vi "Test.vi"() -> ()   [LabVIEW 2016]
uses:
  Globals/PressuresGlobal.vi
  <userlib>/Fluigent/Fluigent MFCS/FluigentMFCS_Full.llb/MFCS_EZ Detect.vi
  <userlib>/Fluigent/Fluigent MFCS/FluigentMFCS_Full.llb/MFCS_EZ Initialization.vi
  <userlib>/Fluigent/Fluigent MFCS/FluigentMFCS_Full.llb/MFCS_EZ Write Channel Pressure.vi
  <vilib>/Utility/file.llb/Write Delimited Spreadsheet (DBL).vi
panel:
  out "Set Pressure Out 2":dbl[](array[numeric])=[825.7187370828326, 752.1790107184136]
  in  "Set Pressure in":dbl[](array[numeric])=[700.0, 700.0]
  out "Set Pressure Out":dbl[](array[numeric])
  in  "file path (dialog if empty)":path=path "E:/maggot images/Jacob/20180102/flow_across_channels_with_same_controller_run101.txt"
  out "Waveform Chart":T1(graph)={"appended array[0]"=534.7139256540268, "appended array[1]"=395.09418314500516}
  in  "Flowboards 2":enum16{"A", "B", "C"}[](array[ring])=[enum."A", enum."A", enum."A", enum."A", enum."B", enum."B"]
  in  "Channels 2":enum16{"1", "2", "3", "4", "5", "6", "7", "8"}[](array[ring])=[enum."1", enum."2", enum."3", enum."4", enum."1", enum."2"]
  in  "Channels":enum16{"1", "2", "3", "4", "5", "6", "7", "8"}[](array[ring])=[enum."1", enum."5"]
  in  "Flowboards":enum16{"A", "B", "C"}[](array[ring])=[enum."A", enum."A"]
  in  "Valve Data":T2
  in  "Water Mix Pressure Channel":i16=2
  in  "Odor Mix Pressure Channel":i16=3
  in  "Ratio":dbl=0.9
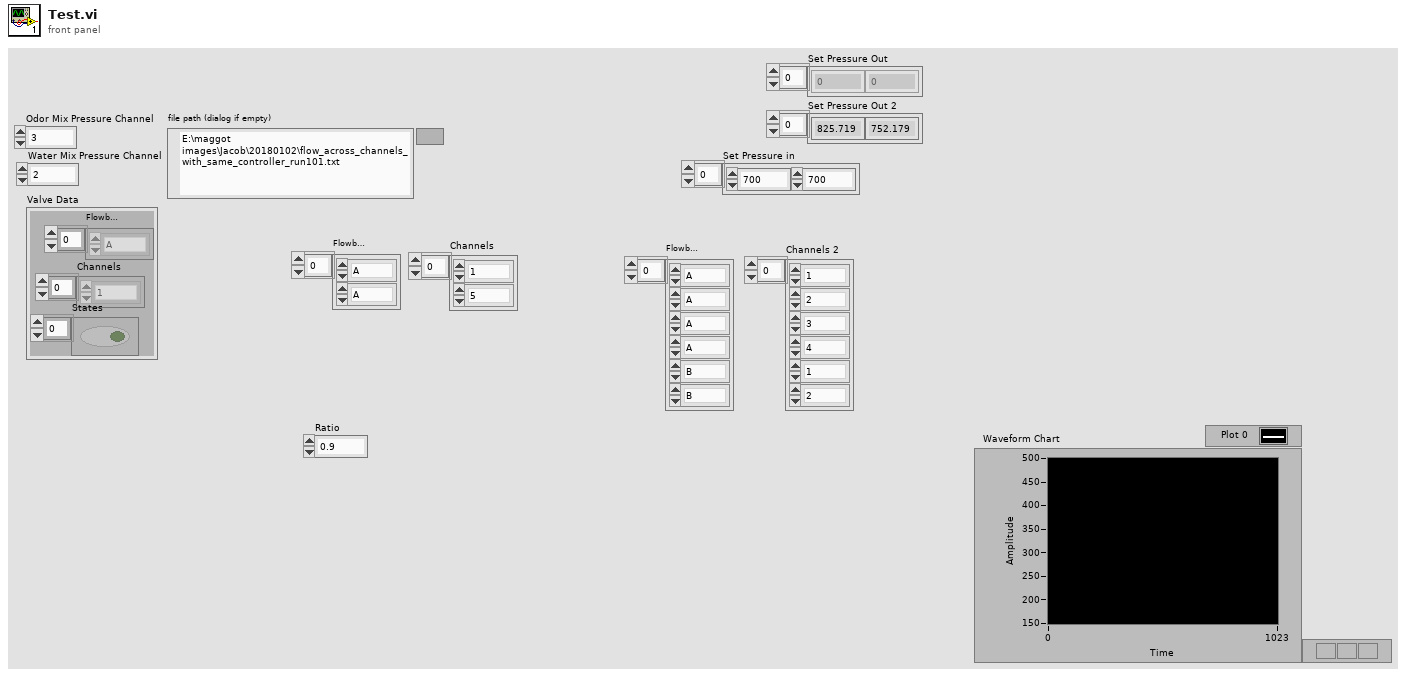
[diagram p1: front panel]
types:
  T1 = cluster{"appended array[0]":dbl, "appended array[1]":dbl}
  T2 = cluster{"Flowboards":enum16{"A", "B", "C"}[], "Channels":enum16{"1", "2", "3", "4", "5", "6", "7", "8"}[], "States":bool[]}
  T3 = enum16{"Release", "Create", "Send", "Wait", "Cancel"}
  T4 = typedef "_EZmfcsSN.ctl" = u16
  T5 = typedef "_EZmfcsRefNum.ctl" = refnum<k1>
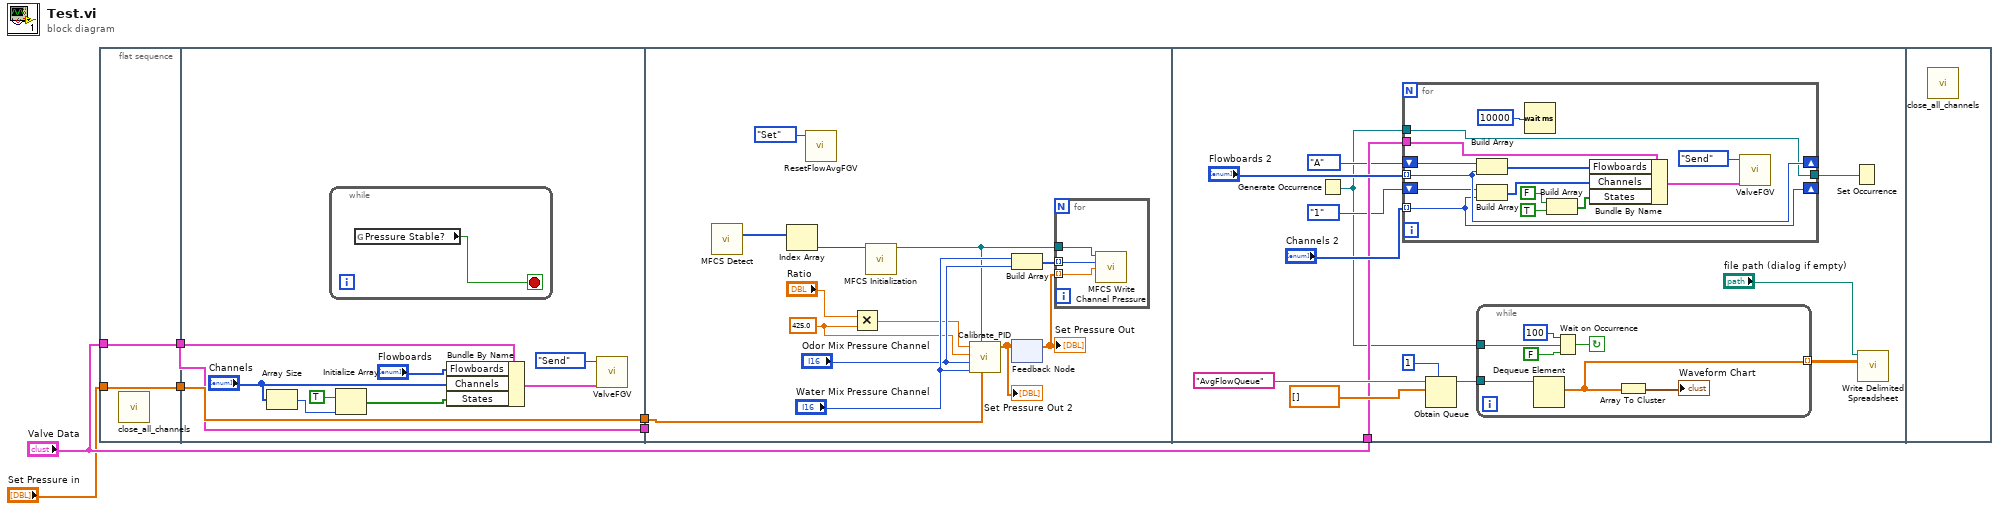
[diagram p0: block diagram]
diagram:
  n1 = flat-sequence {
    tunnel: "Set Pressure in" -> [w7]
    tunnel: "Valve Data" -> [w8]
    tunnel: [w8] -> w4
    tunnel: [w7] -> w2
    tunnel: w4 -> [w12]
    tunnel: [w12] -> w3
    tunnel: w2 -> [w17]
    tunnel: [w17] -> w1
    tunnel: w3 -> [_]
    tunnel: w1 -> [w20]
    tunnel: "Valve Data" -> [w42]
    frame #0 {
      n2 = call "close_all_channels.vi"() -> ()  [unwired: 12 in]
    }
    frame #1 {
      n3 = Array Size(array="Channels") -> (size(s)=w14:i32)
      n4 = while {
        stop <- w18 stop-if-true
        n5 = global read "PressuresGlobal.vi" "Pressure Stable?"() -> (w18:bool)
      }
      n6 = Initialize Array(TRUE, w14) -> (w9:bool[])
      n7 = Bundle By Name(cluster=w12, "Flowboards"="Flowboards", "Channels"="Channels", "States"=w9) -> (w15:T2)
      n8 = call "ValveFGV.vi"("Valve Data"=w15, "Action"=T3."Send") -> ()  [unwired: 6 in, 4 out]
    }
    frame #2 {
      w26 = 425.0 ("Ftot Setpoint")
      n9 = call-poly <userlib>:"MFCS Detect.vi"() -> ("[SN MFCS_EZ]"=w31:T4[])  [unwired: 14 in, 1 out]
      n10 = Index Array(array=w31) -> (element=w30:T4)  [unwired: 1 in]
      n11 = call "ResetFlowAvgFGV.vi"("Action"=enum16{"Create", "Set", "Wait"}."Set") -> ()  [unwired: 10 in, 1 out]
      n12 = Multiply(x="Ratio", y=w26) -> (x*y=w24:dbl)
      n13 = call-poly <userlib>:"MFCS Initialization.vi"("SN MFCS_EZ"=w30) -> ("MFCS_EZ"=w23:T5)  [unwired: 12 in, 2 out]
      n14 = call "Calibrate_PID.vi"("Starting Pressure"=w20, "MFCS_EZ"=w23, "Water Mix Pressure Channel"="Water Mix Pressure Channel", "Odor Mix Pressure Channel"="Odor Mix Pressure Channel", "Ftot Setpoint"=w26, "F1 Setpoint"=w24) -> ("Set Pressure Out"=w22:dbl[])  [unwired: 4 in, 1 out]
      "Set Pressure Out 2" <- w22
      n15 = Build Array("Water Mix Pressure Channel", "Odor Mix Pressure Channel") -> (w27:i16[])
      n16 = feedback-in #1(w22) -> ()
      n17 = feedback #1() -> (w21:dbl[])  [unwired: 1 in]
      "Set Pressure Out" <- w21
      n18 = for {
        tunnel: w21 -> [w34] mode=indexing
        tunnel: w27 -> [w32] mode=indexing
        tunnel: w23 -> [w33]
        n19 = call-poly <userlib>:"MFCS Write Channel Pressure.vi"("MFCS_EZ"=w33, "Channel Number (default=1)"=w32, "Pressure (mBar)"=w34) -> ()  [unwired: 11 in, 2 out]
      }
    }
    frame #3 {
      n20 = Generate Occurrence() -> (w36:refnum<k4>)
      n21 = for {
        tunnel: "Flowboards 2" -> [w64] mode=indexing
        tunnel: "Channels 2" -> [w62] mode=indexing
        tunnel: w42 -> [w68]
        shift-right: [w62] -> _
        shift-left: enum16{"1", "2", "3", "4", "5", "6", "7", "8"}."1" ("Channel") -> [w63]
        shift-right: [w64] -> _
        shift-left: enum16{"A", "B", "C"}."A" ("Flowboard") -> [w65]
        tunnel: w36 -> [w55]
        tunnel: [w55] -> w35
        n22 = Build Array(w65, w64) -> (w67:enum16{"A", "B", "C"}[])
        n23 = Build Array(w63, w62) -> (w66:enum16{"1", "2", "3", "4", "5", "6", "7", "8"}[])
        n24 = Wait (ms)(milliseconds to wait=u32 10000) -> ()  [unwired: 1 out]
        n25 = Build Array(FALSE, TRUE ("element")) -> (w61:bool[])
        n26 = Bundle By Name(cluster=w68, "Flowboards"=w67, "Channels"=w66, "States"=w61) -> (w58:T2)
        n27 = call "ValveFGV.vi"("Valve Data"=w58, "Action"=T3."Send") -> ()  [unwired: 6 in, 4 out]
      }
      n28 = Obtain Queue(max queue size (-1, unlimited)=1, name (unnamed)="AvgFlowQueue", element data type=dbl[] [] ("appended array")) -> (queue out=w39:refnum<queue>)  [unwired: 2 in, 2 out]
      n29 = while {
        tunnel: w39 -> [w54]
        tunnel: [w52] -> w38 mode=indexing
        tunnel: w36 -> [w50]
        stop <- w49 continue-if-true
        n30 = Dequeue Element(queue=w54) -> (element=w52:dbl[])  [unwired: 2 in, 3 out]
        n31 = Wait on Occurrence(1:FALSE ("ignore previous (T)"), 2:w50, 3:u32 100 ("milliseconds to wait")) -> (0:w49:bool)
        n32 = Array To Cluster(array=w52) -> (cluster=→"Waveform Chart":T1)
      }
      n33 = Set Occurrence(w35) -> ()
      n34 = call-poly <vilib>:"Write Delimited Spreadsheet.vi"("file path (dialog if empty)"="file path (dialog if empty)", "2D data"=w38) -> ()  [unwired: 12 in, 2 out]
    }
    frame #4 {
      n35 = call "close_all_channels.vi"() -> ()  [unwired: 12 in]
    }
  }
